vi "Deserialize Core.vi"(8 "error in (no error)":errorcluster, 10 "Serialized Attributes":string, 11 "Serialize in":refnum<class "Serializable Msg.lvclass">) -> (0 "error out":errorcluster, 3 "Serialize out":refnum<class "Serializable Msg.lvclass">)   [LabVIEW 2020, in "Serializer.lvlib" / "Serializable Message.lvlib" / "Serializable Msg.lvclass"]
uses:
  Serializable Msg.lvclass
  Serializable Msg.lvclass/Serializable Msg.ctl
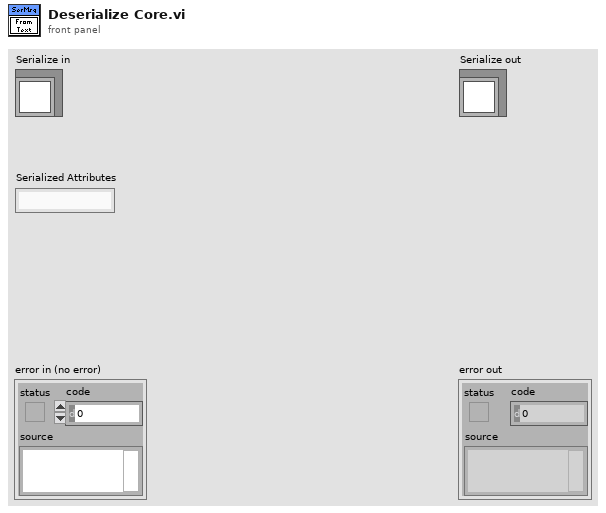
[diagram p1: front panel]
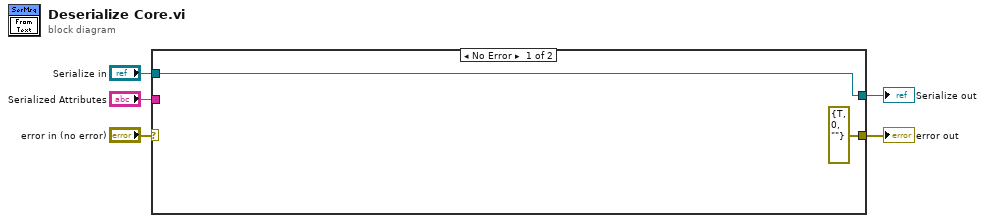
[diagram p0: block diagram]
diagram:
  n1 = case shown="No Error" "error in (no error)" {
    selector: "error in (no error)" -> [_ w9]
    tunnel: [errorcluster {"status"=TRUE, "code"=0, "source"=""} ("error IO") w9] -> w4
    tunnel: "Serialize in" -> [w7 w8]
    tunnel: "Serialized Attributes" -> [_ _]
    tunnel: [w7 w8] -> w1
    frame No Error {
    }
    frame Error {
    }
  }
  "error out" <- w4
  "Serialize out" <- w1
